vi "BuildLabelString.vi"(5 "Y":dbl[](array[numeric]), 6 "Axes":enum16{"Focus only", "X, Y, and focus"}(ring), 7 "X":dbl[](array[numeric]), 8 "error in (no error)":errorcluster, 9 "Image time":dbl, 10 "Focus":dbl[](array[numeric]), 11 "Time array":dbl[](array[numeric])) -> (0 "error out":errorcluster, 3 "Label string":string)   [LabVIEW 2012]
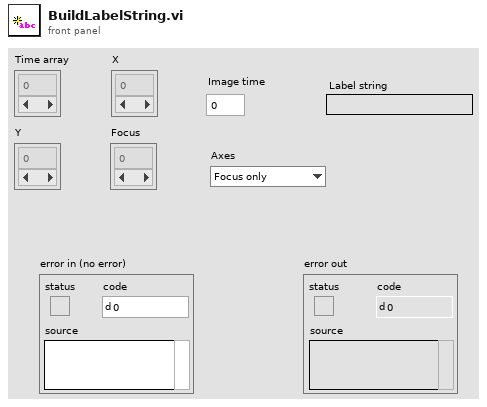
[diagram p1: front panel]
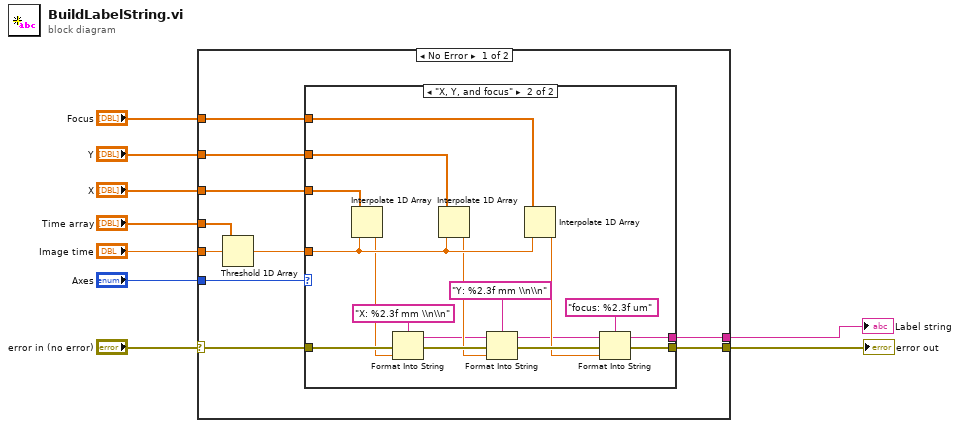
[diagram p0: block diagram]
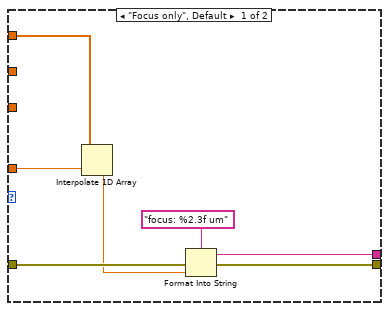
[diagram p2: hidden frame]
diagram:
  n1 = case shown="No Error" "error in (no error)" {
    selector: "error in (no error)" -> [w12 w44]
    tunnel: "Time array" -> [w19 _]
    tunnel: "Image time" -> [w18 _]
    tunnel: "Axes" -> [w17 _]
    tunnel: "X" -> [w15 _]
    tunnel: "Y" -> [w14 _]
    tunnel: "Focus" -> [w13 _]
    tunnel: [w11 w44] -> w2
    tunnel: [w10 _] -> w1
    frame No Error {
      n2 = Threshold 1D Array(2:w18, 3:w19) -> (0:w16:dbl)  [unwired: 1 in]
      n3 = case shown="\"X, Y, and focus\"" w17 {
        tunnel: w16 -> [w26 w43]
        tunnel: w15 -> [_ w42]
        tunnel: w14 -> [_ w41]
        tunnel: w13 -> [w25 w40]
        tunnel: w12 -> [w24 w39]
        tunnel: [w23 w35] -> w11
        tunnel: [w22 w30] -> w10
        frame "Focus only", Default {
          n4 = Interpolate 1D Array(1:w26, 2:w25) -> (0:w21:dbl)
          n5 = Format Into String(format string="focus: %2.3f um", error in=w24, w21) -> (resulting string=w22:string, error out=w23:errorcluster)  [unwired: 1 in]
        }
        frame "X, Y, and focus" {
          n6 = Interpolate 1D Array(1:w43, 2:w42) -> (0:w38:dbl)
          n7 = Format Into String(format string="X: %2.3f mm \\n\\n", error in=w39, w38) -> (resulting string=w32:string, error out=w37:errorcluster)  [unwired: 1 in]
          n8 = Interpolate 1D Array(1:w43, 2:w41) -> (0:w34:dbl)
          n9 = Format Into String(format string="Y: %2.3f mm \\n\\n", initial string=w32, error in=w37, w34) -> (resulting string=w31:string, error out=w36:errorcluster)
          n10 = Interpolate 1D Array(1:w43, 2:w40) -> (0:w33:dbl)
          n11 = Format Into String(format string="focus: %2.3f um", initial string=w31, error in=w36, w33) -> (resulting string=w30:string, error out=w35:errorcluster)
        }
      }
    }
    frame Error {
    }
  }
  "error out" <- w2
  "Label string" <- w1
